vi "TEXT_TO_VOICE.VI"() -> ()   [LabVIEW 2022 SP3]
uses:
  System.Speech
panel:
  in  "?":bool
  in  "String":string
  out "MESSAGE":string="HELLO MASTER VIDWAN"
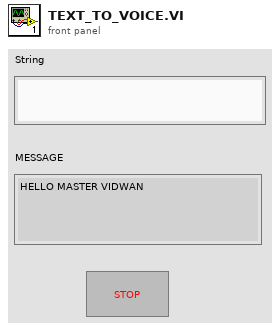
[diagram p1: front panel]
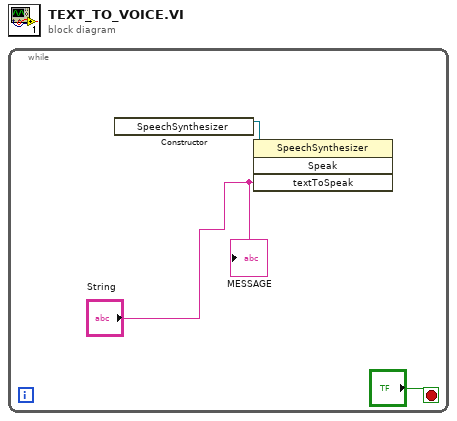
[diagram p0: block diagram]
diagram:
  n1 = while {
    stop <- "?" stop-if-true
    n2 = constructor class="SpeechSynthesizer"() -> (reference out=w3:refnum<k24>)  [unwired: 3 in, 2 out]
    n3 = invoke class="SpeechSynthesizer" method="Speak"(reference=w3, "textToSpeak"="String") -> ()  [unwired: 2 in, 4 out]
    "MESSAGE" <- "String"
  }
